vi "Authorization Global.vi"() -> ()   [LabVIEW 2011]
uses:
  Authorization Data.ctl
panel:
  in  "Authorization":T1
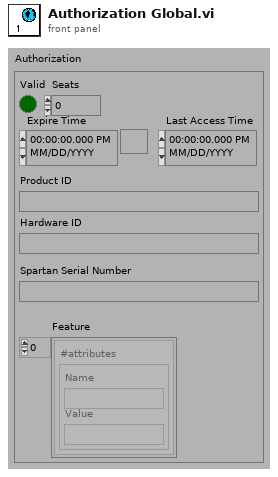
[diagram p1: front panel]
types:
  T1 = typedef "Authorization Data.ctl" = cluster{"Valid":bool, "Seats":i32, "Expire Time":timestamp, "Last Access Time":timestamp, "Product ID":string, "Hardware ID":string, "Spartan Serial Number":string, "Feature":cluster{"#attributes":cluster{"Name":string, "Value":string}}[]}
diagram:
